vi "XNET.CAN.BusMonitor.DiscoveryServer.Execute.vi"(8 "error in (no error)":errorcluster, 11 "CAN.Streaming.API in":refnum<class "XNET.CAN.BusMonitor.API.lvclass">) -> (0 "error out":errorcluster, 3 "CAN.Streaming.API out":refnum<class "XNET.CAN.BusMonitor.API.lvclass">)   [LabVIEW 2025, in "XNET.CAN.BusMonitor.API.lvlib" / "XNET.CAN.BusMonitor.API.lvclass"]
uses:
  XNET.CAN.BusMonitor.API.lvclass
  XNET.CAN.BusMonitor.API.lvclass/XNET.CAN.BusMonitor.API.ctl
  <vilib>/gRPC/LabVIEW gRPC Servicer/ServiceBase/ServiceBase.lvclass
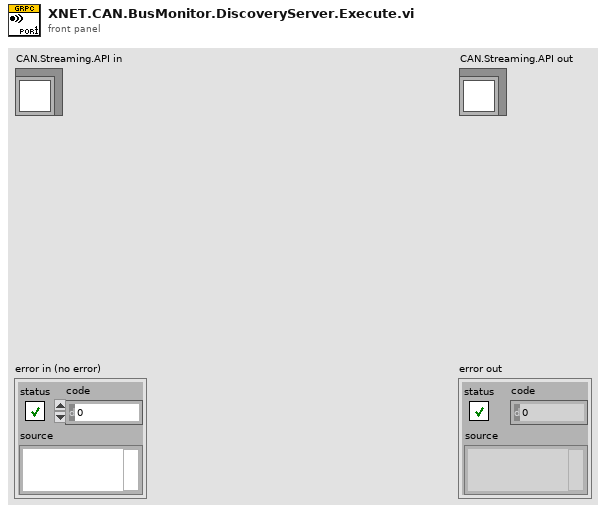
[diagram p1: front panel]
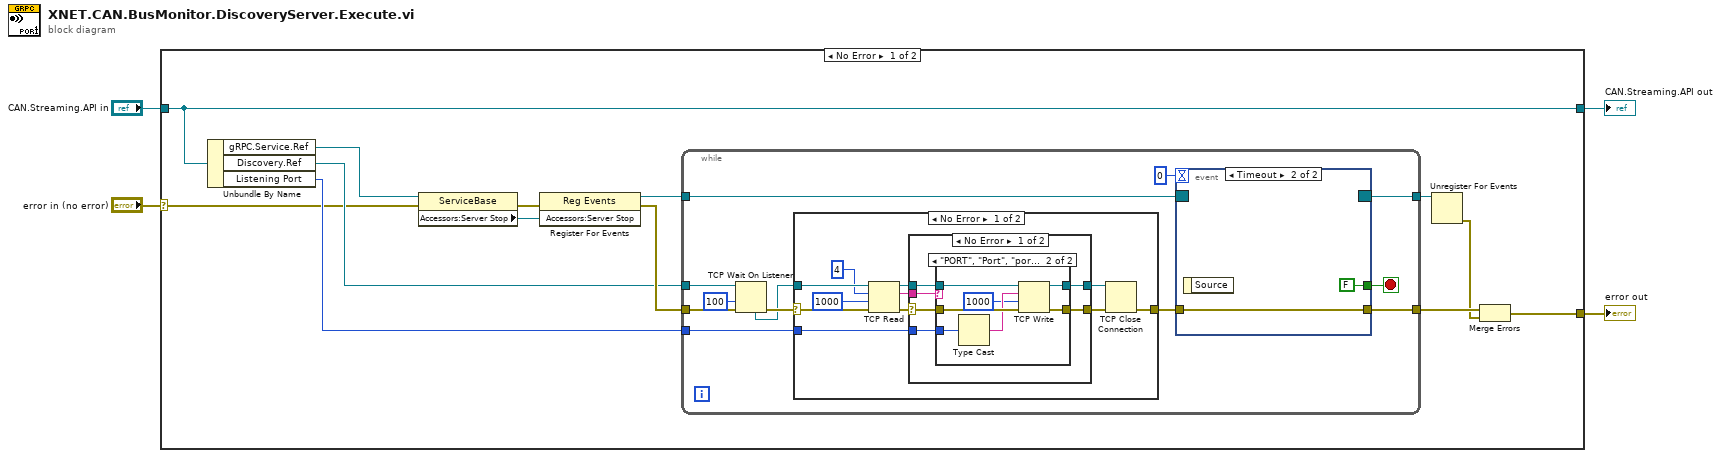
[diagram p0: block diagram]
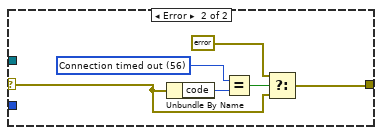
[diagram p4: hidden frame]
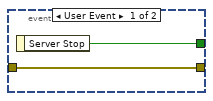
[diagram p5: hidden frame]
diagram:
  n1 = case shown="No Error" "error in (no error)" {
    selector: "error in (no error)" -> [w6 w69]
    tunnel: [w5 w69] -> w3
    tunnel: [w9 w68] -> w1
    tunnel: "CAN.Streaming.API in" -> [w9 w68]
    frame No Error {
      n2 = Unbundle By Name(w9) -> ("gRPC.Service.Ref"=w13:refnum<class "ServiceBase.lvclass">, "Discovery.Ref"=w12:refnum<k5>, "Listening Port"=w11:i32)
      n3 = property class="ServiceBase"(reference=w13, error in=w6) -> (error out=w15:errorcluster, "Accessors:Server Stop"=w17:refnum<user-event>)  [unwired: 1 out]
      n4 = register-events(error in=w15, w17) -> (reference out=w16:refnum<event-registration>, error out=w14:errorcluster)  [unwired: 1 in]
      n5 = while {
        tunnel: w14 -> [w29]
        tunnel: w12 -> [w28]
        tunnel: [w22] -> w8
        tunnel: w16 -> [w20]
        tunnel: w11 -> [w19]
        tunnel: [w18] -> w10
        stop <- w21 stop-if-true
        n6 = TCP Wait On Listener(8:w29, 9:100 ("timeout ms (wait forever: -1)"), 11:w28) -> (0:w26:errorcluster, 4:w25:refnum<k5>)  [unwired: 1 in, 3 out]
        n7 = case shown="No Error" w26 {
          selector: w26 -> [w35 w59]
          tunnel: w25 -> [w40 _]
          tunnel: [w36 w60] -> w23
          tunnel: w19 -> [w30 _]
          frame No Error {
            n8 = TCP Read(connection ID=w40, bytes to read=4, error in (no error)=w35, 9:1000 ("timeout ms (25000)")) -> (connection ID out=w39:refnum<k5>, data out=w32:string, error out=w31:errorcluster)  [unwired: 1 in]
            n9 = case shown="No Error" w31 {
              selector: w31 -> [w42 w56]
              tunnel: w39 -> [w46 w57]
              tunnel: [w45 w57] -> w38
              tunnel: [w44 w56] -> w37
              tunnel: w32 -> [w43 _]
              tunnel: w30 -> [w41 _]
              frame No Error {
                n10 = case shown="\"PORT\", \"Port\", \"port\"" w43 {
                  tunnel: w46 -> [w48 w55]
                  tunnel: [w48 w54] -> w45
                  tunnel: [w47 w53] -> w44
                  tunnel: w42 -> [w47 w52]
                  tunnel: w41 -> [_ w49]
                  frame Default {
                  }
                  frame "PORT", "Port", "port" {
                    n11 = Type Cast(x=w49) -> (*(type *) &x=w51:string)  [unwired: 1 in]
                    n12 = TCP Write(connection ID=w55, data in=w51, error in (no error)=w52, 9:1000 ("timeout ms (25000)")) -> (connection ID out=w54:refnum<k5>, error out=w53:errorcluster)  [unwired: 1 out]
                  }
                }
              }
              frame Error {
              }
            }
            n13 = TCP Close Connection(connection ID=w38, error in (no error)=w37) -> (error out=w36:errorcluster)  [unwired: 1 in, 1 out]
          }
          frame Error {
            w58 = 56 items=["No Error", "Argument Error", "Memory Full", "Out of Zone", "End of File", "File Already Open", "Generic File IO Error", "File Not Found", "File Permission Error", "Disk Full", "Duplicate Path", "Too Many Files Open", "Not Enabled", "Resource File Not Found", "Cannot Add Resource", "Resource Not Found", "Image Not Found", "Image Memory Error", "Pen Does Not Exist", "Config Bad Type", "Config Token Not Found", "Config Parse Error", "Config Memory Error", "Bad External Code Format", "Bad External Code Offset", "External Code Not Present", "Null Window", "Destroy Window Mixup", "Null Menu", "Print Aborted", "Bad Print Record", "Print Driver Error", "Windows Error During Print", "Memory Error During Print", "Print Dialog Error", "Generic Print Error", "Invalid Device Refnum", "Device Not Found", "Device Parameter Error", "Device Unit Error", "Can't Open Device", "Device Call Aborted", "Generic Error", "Cancelled By User", "Object ID Too Low", "Object ID Too High", "Object Not In Heap", "Unknown Heap", "Bad DefProc ID", "DefProc Not In Table", "Message Out Of Range", "Null Method", "Unknown Message", "Manager Call Not Supported", "Bad address", "Connection In progress", "Connection timed out", "Connection is already in progress", "Network attribute not supported", "Network error", "Address in use", "System out of memory", "Connection aborted", "Connection refused", "Connection is not connected", "Connection is already connected", "Connection closed", "Initialize error (interapplication manager)", "Bad occurrence", "Wait on unbound occurrence handler", "Occurrence queue overflow", "Bad path", "Semaphore not signaled", "Unrecognized type (interapplication manager)"] ("1st Error to Convert")
            n14 = Unbundle By Name(w59) -> ("code"=w62:i32)
            n15 = Equal?(x=w58, y=w62) -> (x = y?=w63:bool)
            n16 = Select(t=errorcluster {"status"=FALSE, "code"=0, "source"=""} ("error in (no error)"), s=w63, f=w59) -> (s? t:f=w60:errorcluster)
          }
        }
        n17 = event shown="[1] Timeout" {
          selector: w20 -> [_ _]
          dyn-events: [_ _] -> w18
          timeout: 0 -> [_ _]
          tunnel: [w65 w67] -> w22
          tunnel: w23 -> [w65 w67]
          tunnel: [w64 FALSE ("Server Stop")] -> w21
          event User Event {
            n18 = event-data() -> ("Server Stop"=w64:bool)  [unwired: 1 in]
          }
          event Timeout {
            n19 = event-data() -> ()  [unwired: 1 in, 1 out]
          }
        }
      }
      n20 = Unregister For Events(event registration refnum=w10) -> (error out=w7:errorcluster)  [unwired: 1 in]
      n21 = Merge Errors(w8, w7) -> (w5:errorcluster)
    }
    frame Error {
    }
  }
  "error out" <- w3
  "CAN.Streaming.API out" <- w1
